vi "Find the closest value and index.vi"(5 "Target Value":dbl, 6 "Data":dbl[](array[numeric])) -> (1 "Closest Index of Value":i32, 2 "Closest Value":dbl)   [LabVIEW 2014]
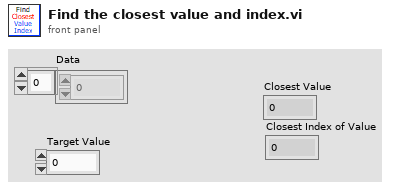
[diagram p1: front panel]
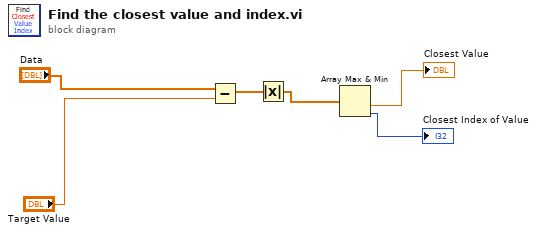
[diagram p0: block diagram]
diagram:
  n1 = Subtract(x="Data", y="Target Value") -> (x-y=w4:dbl[])
  n2 = Absolute Value(x=w4) -> (abs(x)=w3:dbl[])
  n3 = Array Max & Min(array=w3) -> (min value=→"Closest Value":dbl, min index (indices)=→"Closest Index of Value":i32)  [unwired: 2 out]
